vi "Set Step Size Delay.vi"(8 "error in (no error)":errorcluster, 9 "Step Size Delay (0) [s]":dbl format="%#_12g", 10 "Channel (T0)":T1 items=["T0", "T1", "A", "B", "C", "D", "E", "F", "G", "H"], 11 "VISA resource name":refnum<visa-resource-name>) -> (0 "error out":errorcluster, 3 "VISA resource name out":refnum<visa-resource-name>, 4 "Device Errors":cluster{"code":i32, "Text":string}[](array[cluster]))   [LabVIEW 2014, in "Stanford Research DG645 - Driver.lvlib"]
doc: "Delay and Output Command: SSDL c,t\nInstrument Error Check\n\nSet the step size of the delay for channel c to t (in seconds)."
uses:
  Stanford Research DG645 - Driver.lvlib
  Channel.ctl
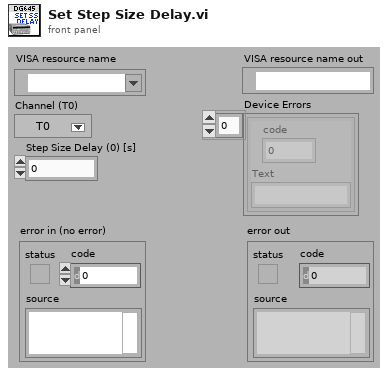
[diagram p1: front panel]
types:
  T1 = typedef "Stanford Research DG645 - Driver.lvlib/Channel.ctl" = i32
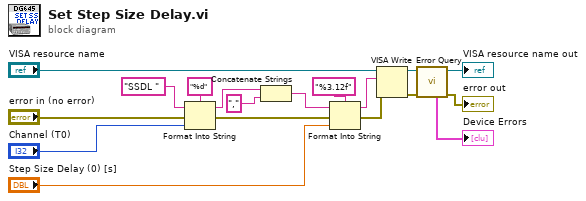
[diagram p0: block diagram]
diagram:
  n1 = Format Into String(format string="%d", initial string="SSDL " ("command"), error in="error in (no error)", "Channel (T0)") -> (resulting string=w16:string, error out=w1:errorcluster)
  n2 = Concatenate Strings(w16, "," ("command")) -> (w2:string)
  n3 = Format Into String(format string="%3.12f", initial string=w2, error in=w1, "Step Size Delay (0) [s]") -> (resulting string=w11:string, error out=w8:errorcluster)
  n4 = VISA Write(VISA resource name="VISA resource name", write buffer=w11, error in (no error)=w8) -> (VISA resource name out=w9:refnum<visa-resource-name>, error out=w5:errorcluster)  [unwired: 1 out]
  n5 = call "Error Query.vi"("error in (no error)"=w5, "VISA resource name"=w9) -> ("error out"=→"error out":errorcluster, "VISA resource name out"=→"VISA resource name out":refnum<visa-resource-name>, "Device Errors"=→"Device Errors":cluster{"code":i32, "Text":string}[])  [unwired: 7 in]
